vi "Auto_One_Ball.vi"() -> ()   [LabVIEW 2015]
panel:
  in  "Clear Error":bool
  in  "To Distance":bool
  out "Rest_Encoder":bool
  out "Rest_Gyro":bool
  in  "Enable":bool
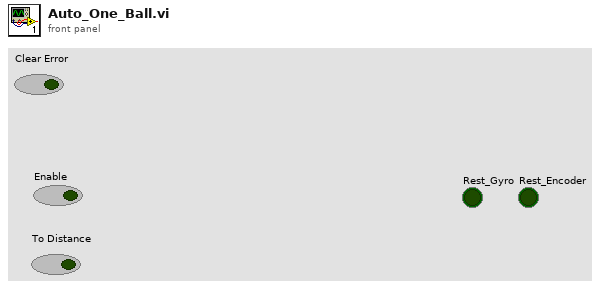
[diagram p1: front panel]
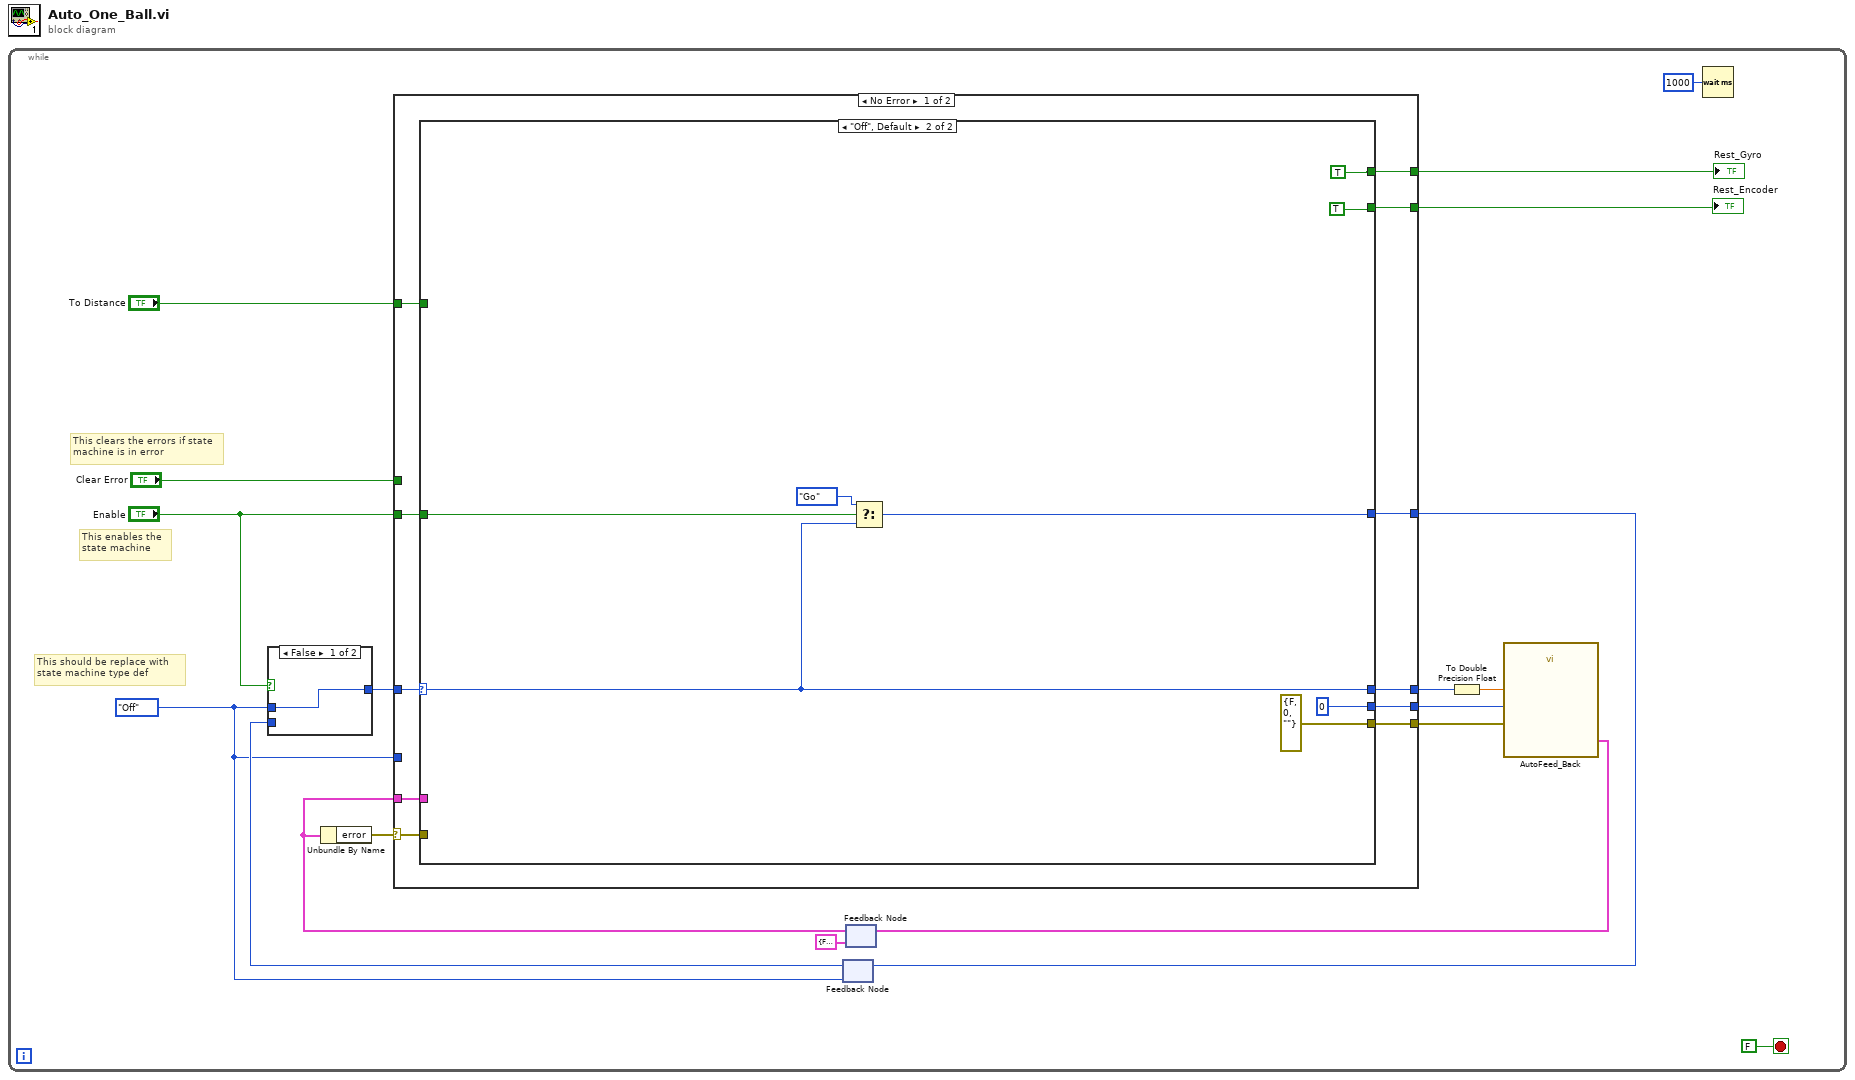
[diagram p0: block diagram]
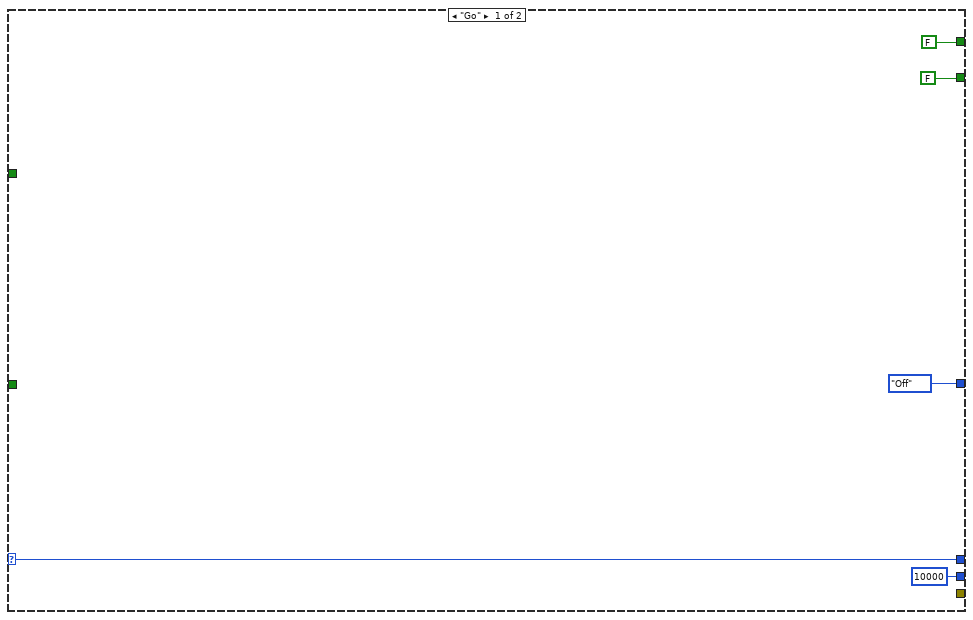
[diagram p3: hidden frame]
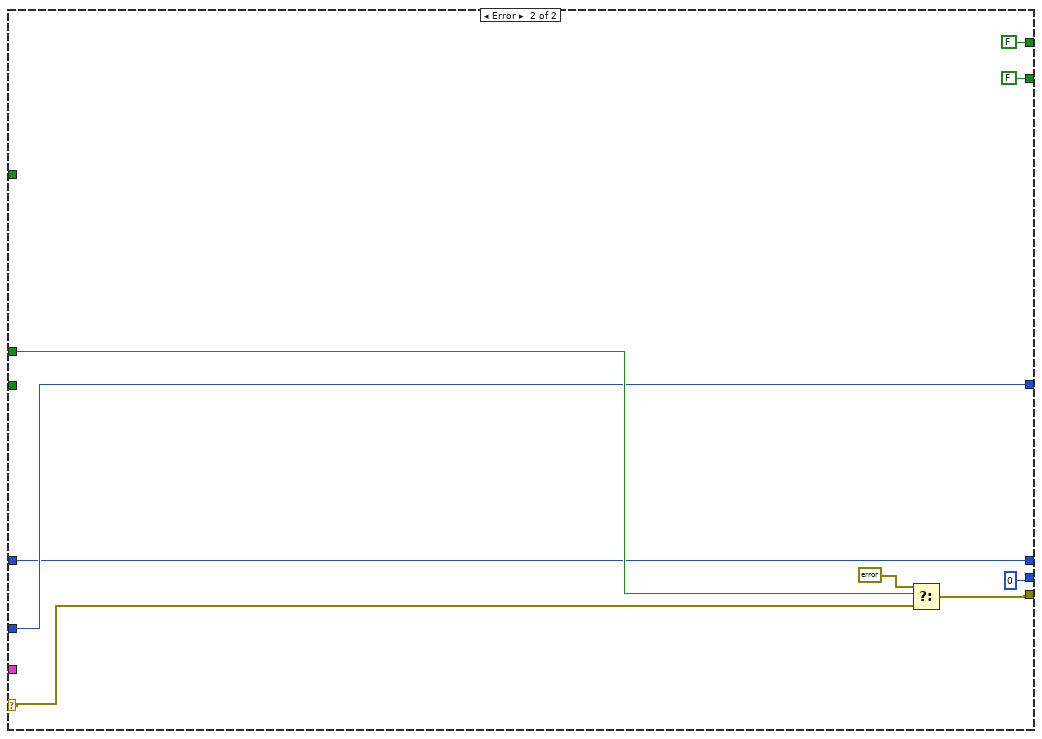
[diagram p4: hidden frame]
diagram:
  n1 = while {
    stop <- FALSE stop-if-true
    w3 = enum16{"Go", "Off"}."Off"
    # "This clears the errors if state \nmachine is in error"
    # "This enables the \nstate machine"
    # "This should be replace with \nstate machine type def"
    n2 = feedback #1(w3) -> (w4:enum16{"Go", "Off"})
    n3 = case shown="False" "Enable" {
      tunnel: w3 -> [w20 _]
      tunnel: [w20 w21] -> w5
      tunnel: w4 -> [_ w21]
      frame False {
      }
      frame True {
      }
    }
    n4 = feedback #2(cluster{"Time_Met":bool, "error ":errorcluster} {"Time_Met"=FALSE, "error "={"status"=FALSE, "code"=0, "source"=""}} ("Feedback_State")) -> (w7:cluster{"Time_Met":bool, "error ":errorcluster})
    n5 = Unbundle By Name(w7) -> ("error"=w9:errorcluster)
    n6 = case shown="No Error" w9 {
      selector: w9 -> [w24 w50]
      tunnel: [w32 FALSE] -> w19
      tunnel: [w31 FALSE] -> w18
      tunnel: "To Distance" -> [w30 _]
      tunnel: [w29 w47] -> w16
      tunnel: [w28 w46] -> w2
      tunnel: [w27 0] -> w13
      tunnel: [w26 w51] -> w12
      tunnel: "Clear Error" -> [_ w49]
      tunnel: w7 -> [w25 _]
      tunnel: "Enable" -> [w23 _]
      tunnel: w5 -> [w22 w46]
      tunnel: w3 -> [_ w47]
      frame No Error {
        n7 = case shown="\"Off\", Default" w22 {
          selector: w22 -> [w35 w40]
          tunnel: [FALSE TRUE] -> w32
          tunnel: [FALSE TRUE] -> w31
          tunnel: [w35 w40] -> w28
          tunnel: [10000 0] -> w27
          tunnel: [enum16{"Go", "Off"}."Off" w39] -> w29
          tunnel: w30 -> [_ _]
          tunnel: [_ errorcluster {"status"=FALSE, "code"=0, "source"=""} ("error")] -> w26
          tunnel: w25 -> [_ _]
          tunnel: w24 -> [_ _]
          tunnel: w23 -> [_ w41]
          frame "Go" {
          }
          frame "Off", Default {
            n8 = Select(t=enum16{"Go", "Off"}."Go", s=w41, f=w40) -> (s? t:f=w39:enum16{"Go", "Off"})
          }
        }
      }
      frame Error {
        n9 = Select(t=errorcluster {"status"=FALSE, "code"=0, "source"=""}, s=w49, f=w50) -> (s? t:f=w51:errorcluster)
      }
    }
    "Rest_Gyro" <- w19
    "Rest_Encoder" <- w18
    n10 = feedback-in #1(w16) -> ()
    n11 = To Double Precision Float(number=w2) -> (double precision float=w1:dbl)
    n12 = call "AutoFeed_Back.vi"("error"=w12, "Time (ms)"=w13, "State"=w1) -> ("Feedback_State"=w11:cluster{"Time_Met":bool, "error ":errorcluster})  [unwired: 8 in]
    n13 = feedback-in #2(w11) -> ()
    n14 = Wait (ms)(milliseconds to wait=u32 1000) -> ()  [unwired: 1 out]
  }
